vi "CetoniPump_Init.vi"(0 "object in":refnum<class "CetoniPump.lvclass">, 2 "Device Configuration Path":string="C:\\Users\\Public\\Documents\\QmixElements\\Projects\\default_project\\Configurations\\sinle", 5 "error in (no error)":errorcluster) -> (14 "object out":refnum<class "CetoniPump.lvclass">, 19 "error out":errorcluster)   [LabVIEW 2021, in "CetoniPump.lvclass"]
uses:
  CetoniPump.lvclass
  CetoniPump.lvclass/CetoniPump.ctl
  Users/olaja/AppData/Local/CETONI_SDK/lib/labview/labbCAN_Bus_API/SiUnitPrefix.ctl
  Users/olaja/AppData/Local/CETONI_SDK/lib/labview/labbCAN_Pump_API/VolumeUnits.ctl
  Users/olaja/AppData/Local/CETONI_SDK/lib/labview/labbCAN_Bus_API/TimeUnits.ctl
  Users/olaja/AppData/Local/CETONI_SDK/lib/labview/labbCAN_Bus_API/labbCAN_Bus_API.lvlib
  Users/olaja/AppData/Local/CETONI_SDK/lib/labview/labbCAN_Pump_API/labbCAN_Pump_API.lvlib
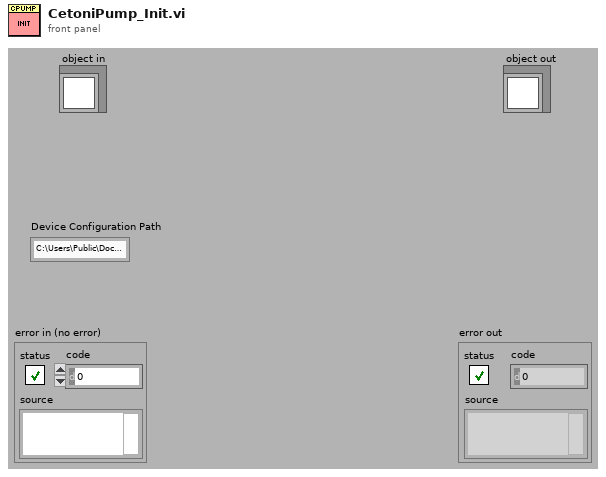
[diagram p1: front panel]
types:
  T1 = cluster{"Pump Handle":i64, "Pump Name":string, "Maximum Volume":dbl, "Maximum Flow Rate":dbl, "Flow Rate":dbl, "Target Level":dbl}[]
  T2 = cluster{"Pump Handle":i64, "Pump Name":string, "Maximum Volume":dbl, "Maximum Flow Rate":dbl, "Flow Rate":dbl, "Target Level":dbl}
  T3 = typedef "labbCAN_Bus_API.lvlib/TimeUnits.ctl" = i32
  T4 = typedef "labbCAN_Pump_API.lvlib/VolumeUnits.ctl" = i32
  T5 = typedef "labbCAN_Bus_API.lvlib/SiUnitPrefix.ctl" = i32
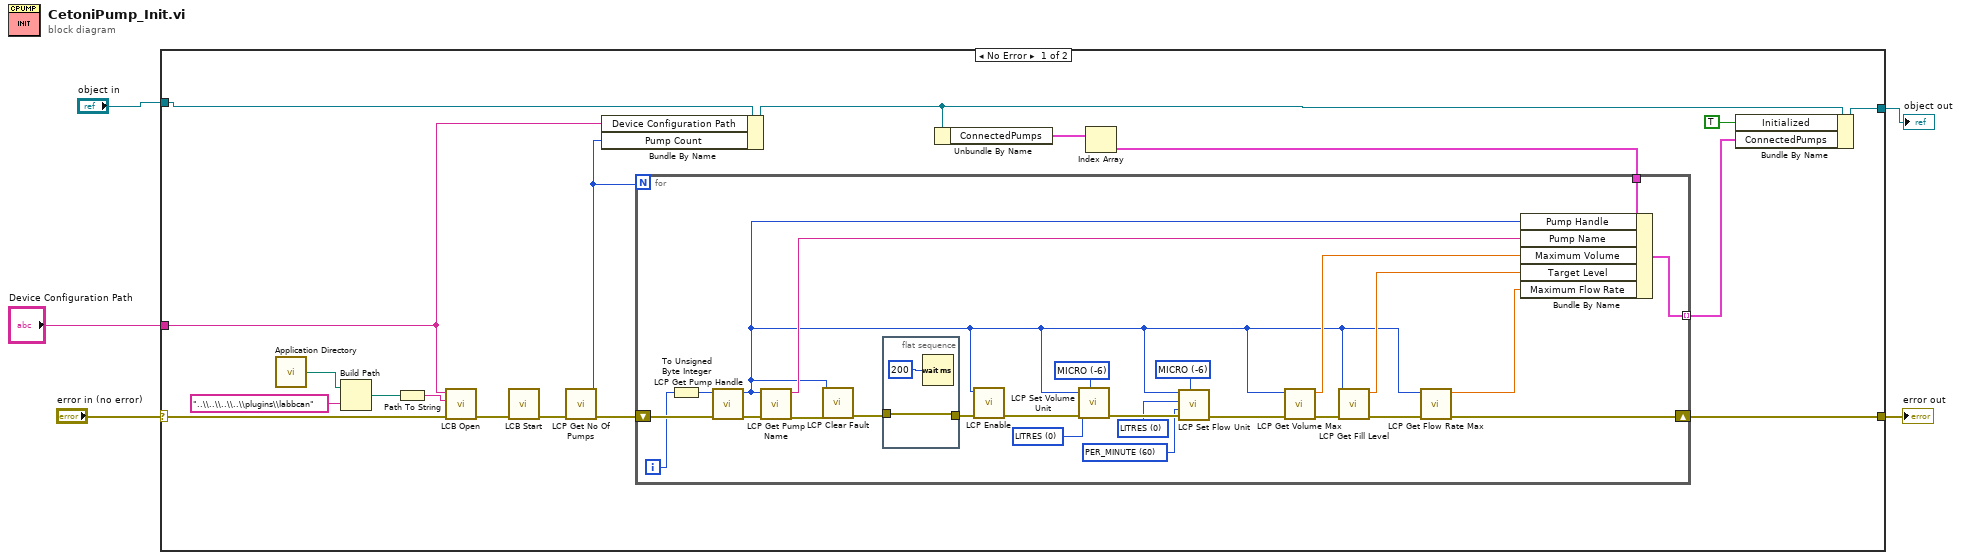
[diagram p0: block diagram]
diagram:
  n1 = case shown="No Error" "error in (no error)" {
    selector: "error in (no error)" -> [w18 w51]
    tunnel: "object in" -> [w23 w52]
    tunnel: [w16 w52] -> w4
    tunnel: [w15 w51] -> w2
    tunnel: "Device Configuration Path" -> [w17 _]
    frame No Error {
      n2 = call <vilib>:"Application Directory.vi"() -> ("Application Directory"=w22:path)
      n3 = Build Path(base path=w22, name or relative path="..\\..\\..\\..\\plugins\\labbcan" ("Name oder relativer Pfad")) -> (appended path=w21:path)
      n4 = Path To String(path=w21) -> (string=w20:string)
      n5 = call "LCB Open.vi"("error in (no error)"=w18, "PluginSearchPath"=w20, "Device Configuration Path"=w17) -> ("error out"=w12:errorcluster)  [unwired: 8 in]
      n6 = call "LCB Start.vi"("error in (no error)"=w12) -> ("error out"=w11:errorcluster)  [unwired: 10 in]
      n7 = call "LCP Get No Of Pumps.vi"("error in (no error)"=w11) -> ("error out"=w13:errorcluster, "Pump Count"=w6:i32)  [unwired: 9 in]
      n8 = Bundle By Name(cluster=w23, "Device Configuration Path"=w17, "Pump Count"=w6) -> (w10:refnum<class "CetoniPump.lvclass">)
      n9 = Unbundle By Name(w10) -> ("ConnectedPumps"=w9:T1)
      n10 = Index Array(array=w9) -> (element=w8:T2)  [unwired: 1 in]
      n11 = for {
        N: w6 -> [_]
        shift-right: [w38] -> w15
        shift-left: w13 -> [w37]
        tunnel: w8 -> [w34]
        tunnel: [w31] -> w7 mode=indexing
        i -> [w27]
        w43 = T3 60 items=["PER_SECOND"=1, "PER_MINUTE"=60, "PER_HOUR"=3600] ("TimeUnit")
        w44 = T4 0 items=["LITRES"] ("VolumeUnit")
        w45 = T4 0 items=["LITRES"] ("Volume Unit")
        w46 = T5 -6 items=["UNIT"=0, "DECI"=-1, "CENTI"=-2, "MILLI"=-3, "MICRO"=-6] ("Prefix")
        w48 = T5 -6 items=["UNIT"=0, "DECI"=-1, "CENTI"=-2, "MILLI"=-3, "MICRO"=-6] ("Prefix")
        n12 = To Unsigned Byte Integer(number=w27) -> (unsigned 8bit integer=w26:u8)
        n13 = call "LCP Get Pump Handle.vi"("error in (no error)"=w37, "Pump Index"=w26) -> ("error out"=w36:errorcluster, "Pump Handle"=w25:i64)  [unwired: 8 in]
        n14 = call "LCP Get Pump Name.vi"("error in (no error)"=w36, "Pump Handle"=w25) -> ("error out"=w35:errorcluster, "Pump Name"=w33:string)  [unwired: 8 in]
        n15 = call "LCP Clear Fault.vi"("error in (no error)"=w35, "Pump Handle"=w25) -> ("error out"=w24:errorcluster)  [unwired: 9 in]
        n16 = flat-sequence {
          tunnel: w24 -> [w49]
          tunnel: [w49] -> w28
          frame #0 {
            n17 = Wait (ms)(milliseconds to wait=u32 200) -> ()  [unwired: 1 out]
          }
        }
        n18 = call "LCP Enable.vi"("error in (no error)"=w28, "Pump Handle"=w25) -> ("error out"=w42:errorcluster)  [unwired: 9 in]
        n19 = call "LCP Set Volume Unit.vi"("Prefix"=w48, "error in (no error)"=w42, "Volume Unit"=w45, "Pump Handle"=w25) -> ("error out"=w47:errorcluster)  [unwired: 7 in]
        n20 = call "LCP Set Flow Unit.vi"("Prefix"=w46, "error in (no error)"=w47, "TimeUnit"=w43, "VolumeUnit"=w44, "Pump Handle"=w25) -> ("error out"=w39:errorcluster)  [unwired: 6 in]
        n21 = call "LCP Get Volume Max.vi"("error in (no error)"=w39, "Pump Handle"=w25) -> ("error out"=w41:errorcluster, "Maximum Volume"=w32:dbl)  [unwired: 8 in]
        n22 = call "LCP Get Fill Level.vi"("error in (no error)"=w41, "Pump Handle"=w25) -> ("error out"=w40:errorcluster, "Fill Level"=w29:dbl)  [unwired: 8 in]
        n23 = call "LCP Get Flow Rate Max.vi"("error in (no error)"=w40, "Pump Handle"=w25) -> ("error out"=w38:errorcluster, "Maximum Flow Rate"=w30:dbl)  [unwired: 8 in]
        n24 = Bundle By Name(cluster=w34, "Pump Handle"=w25, "Pump Name"=w33, "Maximum Volume"=w32, "Target Level"=w29, "Maximum Flow Rate"=w30) -> (w31:T2)
      }
      n25 = Bundle By Name(cluster=w10, "Initialized"=TRUE, "ConnectedPumps"=w7) -> (w16:refnum<class "CetoniPump.lvclass">)
    }
    frame Error {
    }
  }
  "object out" <- w4
  "error out" <- w2
